vi "Configure Trigger (Nth Edge).vi"(0 "VISA resource name":refnum<visa-resource-name>, 1 "Idle Time (1E-6 s)":dbl=1e-06, 2 "Trigger Level (0)":dbl, 5 "Source (1: Channel 1)":i32(ring)=1 items=["Channel 1"=1, "Channel 2"=2, "Channel 3"=3, "Channel 4"=4], 9 "Edge Type (0: Positive)":i32(ring) items=["Positive", "Negative"], 11 "error in (no error)":errorcluster, 12 "Edge Number (2)":dbl=2.0) -> (4 "VISA resource name out":refnum<visa-resource-name>, 15 "error out":errorcluster)   [LabVIEW 2015, in "ZhiYuan ZDS Series for TCP.lvlib"]
doc: "Configures the setting for Nth trigger.\n\nNote: This VI is only applicable for DS 2000 Series."
uses:
  ZhiYuan ZDS Series for TCP.lvlib
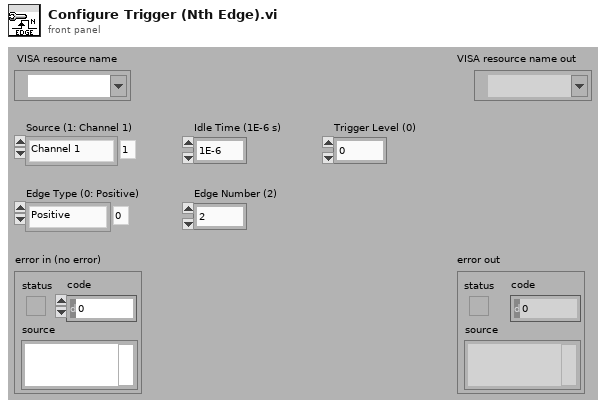
[diagram p1: front panel]
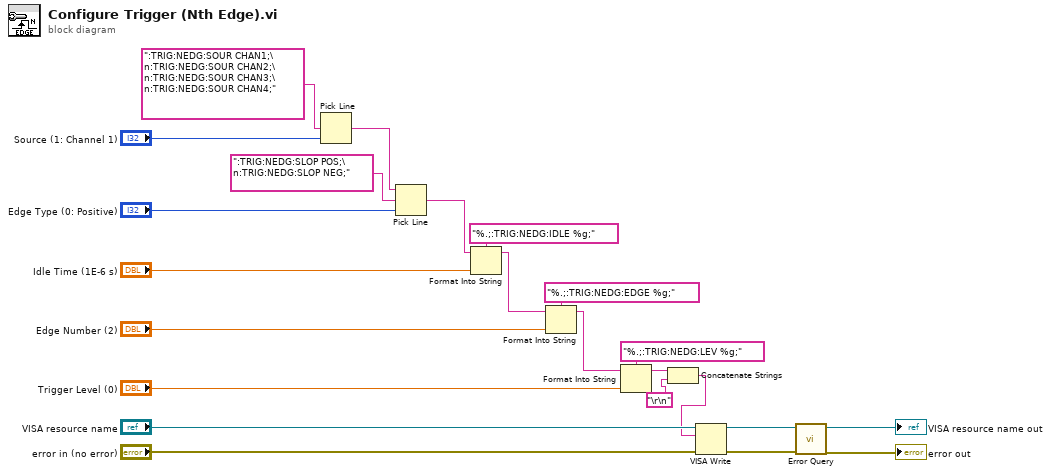
[diagram p0: block diagram]
diagram:
  n1 = Pick Line(multi-line string=":TRIG:NEDG:SOUR CHAN1;\n:TRIG:NEDG:SOUR CHAN2;\n:TRIG:NEDG:SOUR CHAN3;\n:TRIG:NEDG:SOUR CHAN4;", line index="Source (1: Channel 1)") -> (output string=w19:string)  [unwired: 1 in]
  n2 = Pick Line(string ("")=w19, multi-line string=":TRIG:NEDG:SLOP POS;\n:TRIG:NEDG:SLOP NEG;", line index="Edge Type (0: Positive)") -> (output string=w18:string)
  n3 = Format Into String(format string="%.;:TRIG:NEDG:IDLE %g;", initial string=w18, "Idle Time (1E-6 s)") -> (resulting string=w15:string)  [unwired: 1 in, 1 out]
  n4 = Format Into String(format string="%.;:TRIG:NEDG:EDGE %g;", initial string=w15, "Edge Number (2)") -> (resulting string=w12:string)  [unwired: 1 in, 1 out]
  n5 = Format Into String(format string="%.;:TRIG:NEDG:LEV %g;", initial string=w12, "Trigger Level (0)") -> (resulting string=w3:string)  [unwired: 1 in, 1 out]
  n6 = Concatenate Strings(w3, "\r\n") -> (w1:string)
  n7 = VISA Write(VISA resource name="VISA resource name", write buffer=w1, error in (no error)="error in (no error)") -> (VISA resource name out=w7:refnum<visa-resource-name>, error out=w6:errorcluster)  [unwired: 1 out]
  n8 = call "Error Query.vi"("error in (no error)"=w6, "VISA resource name"=w7) -> ("error out"=→"error out":errorcluster, "VISA resource name out"=→"VISA resource name out":refnum<visa-resource-name>)  [unwired: 6 in, 2 out]
